vi "single zip.vi"(8 "error in":errorcluster, 9 "del source?":bool, 10 "source file path":path caption="source path", 11 "comments":string) -> (0 "error out":errorcluster, 2 "output zip":path)   [LabVIEW 2011]
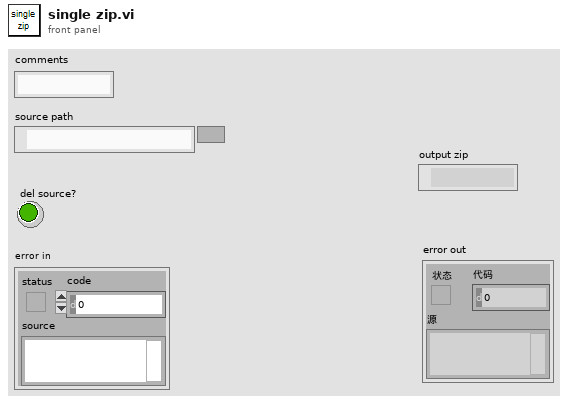
[diagram p1: front panel]
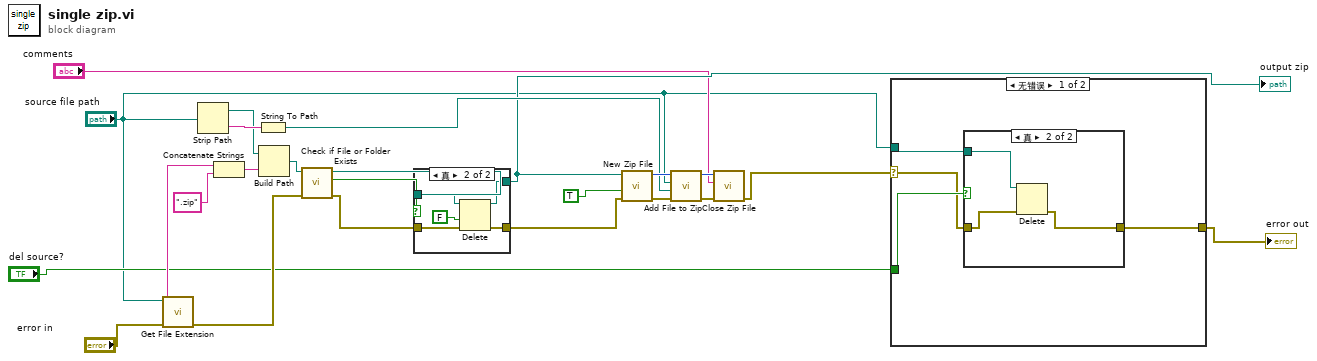
[diagram p0: block diagram]
diagram:
  n1 = call <nishared>:"Get File Extension.vi"("error in (no error)"="error in", "file"="source file path") -> ("error out"=w11:errorcluster, "filename without extension"=w19:string)  [unwired: 6 in, 2 out]
  n2 = Strip Path(path="source file path") -> (stripped path=w16:path, name=w23:string)
  n3 = Concatenate Strings(w19, ".zip" ("字符串")) -> (w17:string)
  n4 = String To Path(string=w23) -> (path=w22:path)
  n5 = Build Path(base path=w16, name or relative path=w17) -> (appended path=w15:path)
  n6 = call <vilib>:"Check if File or Folder Exists.vi"("error in (no error)"=w11, "path"=w15) -> ("error out"=w10:errorcluster, "file or folder exists?"=w5:bool, "dup path"=w14:path)  [unwired: 7 in]
  n7 = case shown="真" w5 {
    tunnel: w14 -> [w26 w31]
    tunnel: [w26 w29] -> w13
    tunnel: w10 -> [w25 w28]
    tunnel: [w25 w27] -> w9
    frame False {
    }
    frame True {
      n8 = Delete(path (use dialog)=w31, confirm (F)=FALSE ("确认(F)"), error in=w28) -> (deleted path=w29:path, error out=w27:errorcluster)  [unwired: 2 in, 1 out]
    }
  }
  "output zip" <- w13
  n9 = call <vilib>:"New Zip File.vi"("error in (no error)"=w9, "confirm overwrite? (F)"=TRUE, "target"=w13) -> ("error out"=w8:errorcluster, "zip file out"=w24:i64)  [unwired: 2 in, 1 out]
  n10 = call <vilib>:"Add File to Zip.vi"("error in (no error)"=w8, "destination path in zip"=w22, "source file path"="source file path", "zip file in"=w24) -> ("error out"=w7:errorcluster, "zip file out"=w20:i64)  [unwired: 6 in]
  n11 = call <vilib>:"Close Zip File.vi"("error in (no error)"=w7, "comments"="comments", "zip file in"=w20) -> ("error out"=w4:errorcluster)  [unwired: 4 in]
  n12 = case shown="无错误" w4 {
    selector: w4 -> [w33 w40]
    tunnel: "del source?" -> [w35 _]
    tunnel: "source file path" -> [w34 _]
    tunnel: [w32 w40] -> w1
    frame No Error {
      n13 = case shown="真" w35 {
        tunnel: w34 -> [_ w39]
        tunnel: w33 -> [w36 w38]
        tunnel: [w36 w37] -> w32
        frame False {
        }
        frame True {
          n14 = Delete(path (use dialog)=w39, error in=w38) -> (error out=w37:errorcluster)  [unwired: 3 in, 2 out]
        }
      }
    }
    frame Error {
    }
  }
  "error out" <- w1
